vi "LCDSetBacklightState.vi"(0 "error in (no error)":errorcluster, 2 "Backlight":dbl, 3 "Device In":u64) -> (7 "error out":errorcluster, 10 "Device Out":u64)   [LabVIEW 2020, in "Phidget LCD.lvlib"]
doc: "${Backlight:Header}"
uses:
  <instrlib>/Phidgets/Phidget LCD/Phidget LCD.lvlib
  <instrlib>/Phidgets/Phidget Common/Phidget Common.lvlib
  phidget22.dll
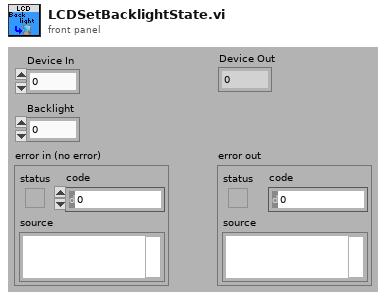
[diagram p1: front panel]
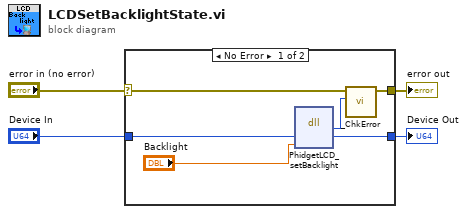
[diagram p0: block diagram]
diagram:
  n1 = case shown="No Error" "error in (no error)" {
    selector: "error in (no error)" -> [w7 w12]
    tunnel: [w6 w12] -> w3
    tunnel: "Device In" -> [w10 w11]
    tunnel: [w9 w11] -> w1
    frame No Error {
      n2 = dll-call lib="phidget22.*" fn="PhidgetLCD_setBacklight"("phid"=w10, "backlight"="Backlight") -> ("return type"=w8:i32, "phid"=w9:u64)  [unwired: 4 in, 2 out]
      n3 = call <instrlib>:"_ChkError.vi"("Return Code"=w8, "error in (no error)"=w7) -> ("error out"=w6:errorcluster)  [unwired: 9 in]
    }
    frame Error {
    }
  }
  "error out" <- w3
  "Device Out" <- w1
